vi "Call Dropsnip.vi"   [LabVIEW 2015]
uses:
  input/input.lvclass
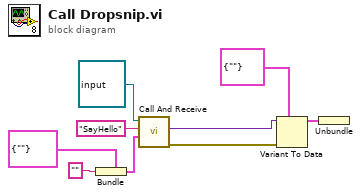
[diagram p0: block diagram]
diagram:
  n1 = Bundle(cluster=cluster{"Greeting":string} {"Greeting"=""}, "Greeting"="") -> (w3:cluster{"Greeting":string})
  n2 = call "Call And Receive.vi"("Parameter"=w3, "Function"="SayHello", "input in"=refnum<class "input.lvclass"> refnum) -> ("error out"=w1:errorcluster, "Data"=w2:variant)  [unwired: 5 in, 2 out]
  n3 = Variant To Data(error in=w1, type=cluster{"Answer":string} {"Answer"=""}, Variant=w2) -> (data=w6:cluster{"Answer":string})  [unwired: 1 out]
  n4 = Unbundle(w6) -> ()  [unwired: 1 out]
